vi "write_data.vi"(8 "error in (no error)":errorcluster, 10 "data":T1={"check_input"=TRUE}, 11 "IncrementalPCA in":refnum<class "IncrementalPCA.lvclass">) -> (0 "error out":errorcluster, 3 "IncrementalPCA out":refnum<class "IncrementalPCA.lvclass">)   [LabVIEW 2020, in "IncrementalPCA.lvclass"]
uses:
  IncrementalPCA.lvclass
  Controls/incremental_pca_data.ctl
  IncrementalPCA.lvclass/IncrementalPCA.ctl
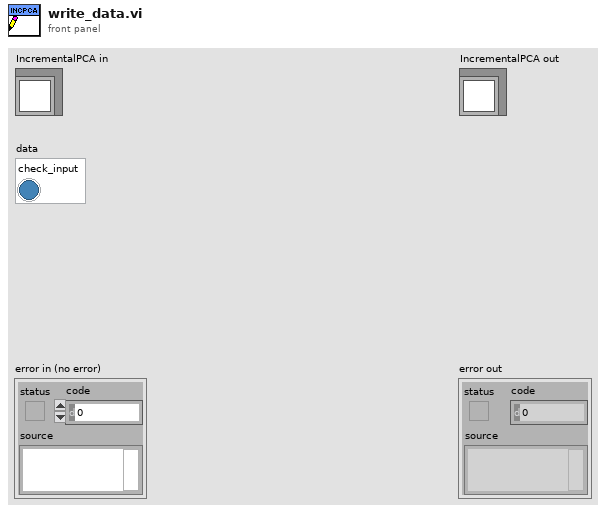
[diagram p1: front panel]
types:
  T1 = typedef "incremental_pca_data.ctl" = cluster{"check_input":bool}
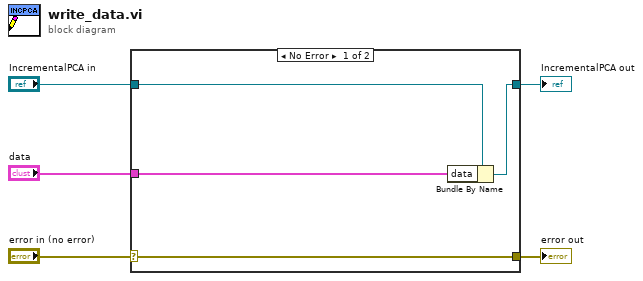
[diagram p0: block diagram]
diagram:
  n1 = case shown="No Error" "error in (no error)" {
    selector: "error in (no error)" -> [w9 w10]
    tunnel: [w9 w10] -> w4
    tunnel: [w7 w11] -> w2
    tunnel: "IncrementalPCA in" -> [w8 w11]
    tunnel: "data" -> [w6 _]
    frame No Error {
      n2 = Bundle By Name(cluster=w8, "data"=w6) -> (w7:refnum<class "IncrementalPCA.lvclass">)
    }
    frame Error {
    }
  }
  "error out" <- w4
  "IncrementalPCA out" <- w2
